vi "set_control_shortcut_menu_item_state.vi"(5 "Checked? (F)":bool, 7 "Enabled? (T)":bool=TRUE, 8 "error in (no error)":errorcluster, 9 "Shortcut":T1, 10 "Item Tag":string, 11 "IControlShortcutMenu In":refnum<class "IControlShortcutMenu.lvclass">) -> (0 "error out":errorcluster, 3 "IControlShortcutMenu Out":refnum<class "IControlShortcutMenu.lvclass">)   [LabVIEW 2015, in "ActorEvents.lvlib" / "IControlShortcutMenu.lvclass"]
uses:
  IControlShortcutMenu.lvclass
  <vilib>/Utility/miscctls.llb/LVMenuShortCut.ctl
panel:
  # "STUB"
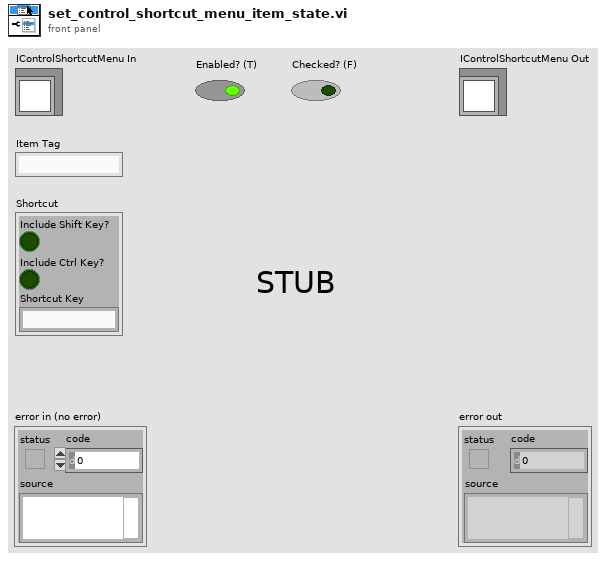
[diagram p1: front panel]
types:
  T1 = typedef "LVMenuShortCut.ctl" = cluster{"Include Shift Key?":bool, "Include Ctrl Key?":bool, "Shortcut Key":string}
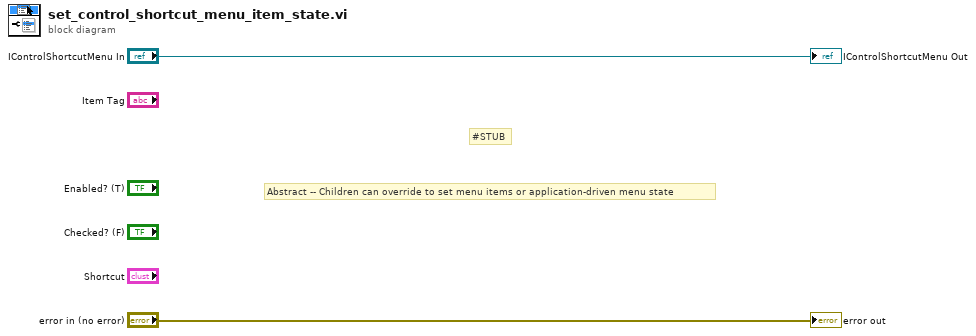
[diagram p0: block diagram]
diagram:
  # "#STUB"
  # "Abstract -- Children can override to set menu items or application-driven menu state"
  "error out" <- "error in (no error)"
  "IControlShortcutMenu Out" <- "IControlShortcutMenu In"
